vi "vacPIDantiWindup.vi"(4 "Saturation U":dbl, 6 "Saturation M":dbl, 7 "Reset":bool, 8 "PID Gains":cluster{"Kp":dbl, "Kd":dbl, "Ki":dbl, "Ts":dbl}={"Kp"=0.0, "Kd"=0.0, "Ki"=0.0, "Ts"=1.0}, 10 "Feedback":dbl, 11 "Reference":dbl) -> (3 "Control":dbl)   [LabVIEW 2016]
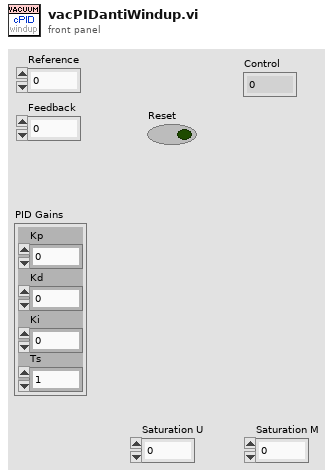
[diagram p1: front panel]
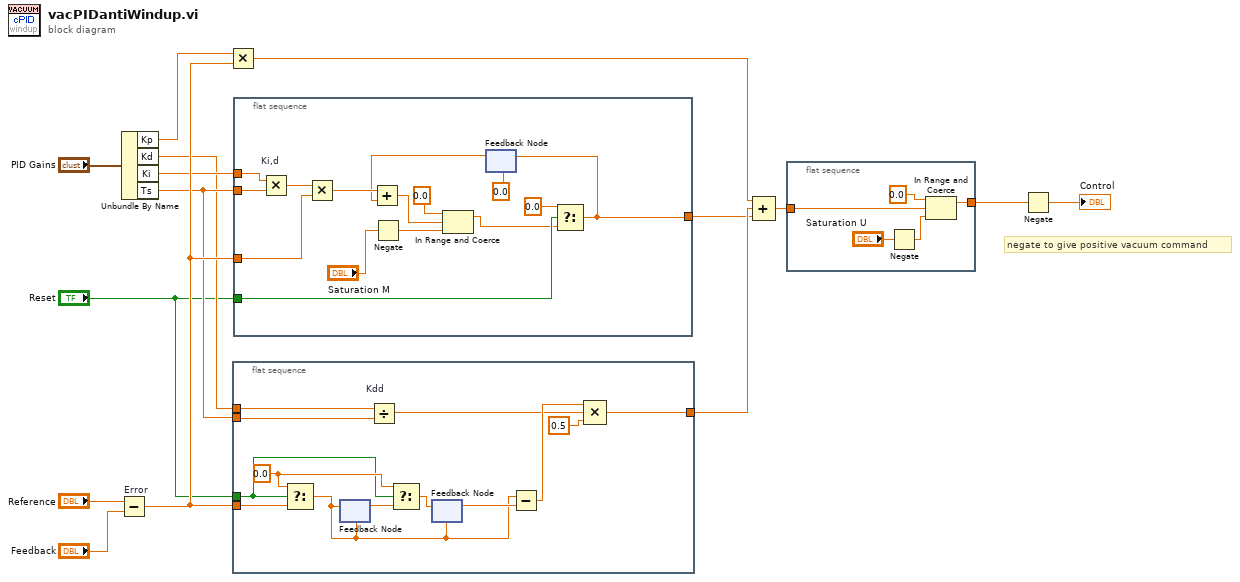
[diagram p0: block diagram]
diagram:
  # "negate to give positive vacuum command"
  n1 = Subtract "Error"(x="Reference", y="Feedback") -> (x-y=w8:dbl)
  n2 = Unbundle By Name("PID Gains") -> ("Kp"=w12:dbl, "Kd"=w5:dbl, "Ki"=w7:dbl, "Ts"=w6:dbl)
  n3 = Multiply(x=w12, y=w8) -> (x*y=w11:dbl)
  n4 = flat-sequence {
    tunnel: [w25] -> w10
    tunnel: w8 -> [w20]
    tunnel: w6 -> [w24]
    tunnel: w5 -> [w23]
    tunnel: "Reset" -> [w16]
    frame #0 {
      w17 = 0.0 ("t")
      n5 = Select(t=w17, s=w16, f=w20) -> (s? t:f=w21:dbl)
      n6 = feedback #1(w21) -> (w19:dbl)
      n7 = feedback-in #1(w21) -> ()
      n8 = Divide "Kdd"(x=w23, y=w24) -> (x/y=w22:dbl)
      n9 = Select(t=w17, s=w16, f=w19) -> (s? t:f=w18:dbl)
      n10 = feedback #2(w21) -> (w28:dbl)
      n11 = feedback-in #2(w18) -> ()
      n12 = Subtract(x=w21, y=w28) -> (x-y=w27:dbl)
      n13 = Compound Arithmetic op=MULTIPLY(w27, w22, 0.5 ("value")) -> (w25:dbl)
    }
  }
  n14 = flat-sequence {
    tunnel: [w30] -> w9
    tunnel: w8 -> [w43]
    tunnel: w7 -> [w41]
    tunnel: w6 -> [w39]
    tunnel: "Reset" -> [w33]
    frame #0 {
      n15 = Multiply "Ki,d"(x=w41, y=w39) -> (x*y=w40:dbl)
      n16 = Multiply(x=w40, y=w43) -> (x*y=w42:dbl)
      n17 = Negate(x="Saturation M") -> (-x=w36:dbl)
      n18 = feedback #3(0.0 ("value")) -> (w34:dbl)
      n19 = Add(x=w42, y=w34) -> (x+y=w38:dbl)
      n20 = In Range and Coerce(upper limit=0.0, x=w38, lower limit=w36) -> (coerced(x)=w32:dbl)  [unwired: 1 out]
      n21 = Select(t=0.0 ("value"), s=w33, f=w32) -> (s? t:f=w30:dbl)
      n22 = feedback-in #3(w30) -> ()
    }
  }
  n23 = Compound Arithmetic op=ADD(w11, w10, w9) -> (w4:dbl)
  n24 = flat-sequence {
    tunnel: w4 -> [w46]
    tunnel: [w45] -> w1
    frame #0 {
      n25 = Negate(x="Saturation U") -> (-x=w47:dbl)
      n26 = In Range and Coerce(upper limit=0.0, x=w46, lower limit=w47) -> (coerced(x)=w45:dbl)  [unwired: 1 out]
    }
  }
  n27 = Negate(x=w1) -> (-x=→"Control":dbl)
